vi "Checksum_example.vi"() -> ()   [LabVIEW 2014]
panel:
  in  "String in 2":string
  in  "String in":string
  out "Match?":bool
  out "Checksum":string
  out "Message":string
  out "Example message":string
  out "Calculated checksum":string
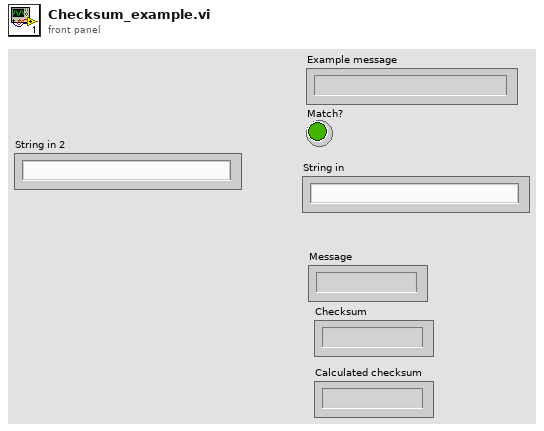
[diagram p1: front panel]
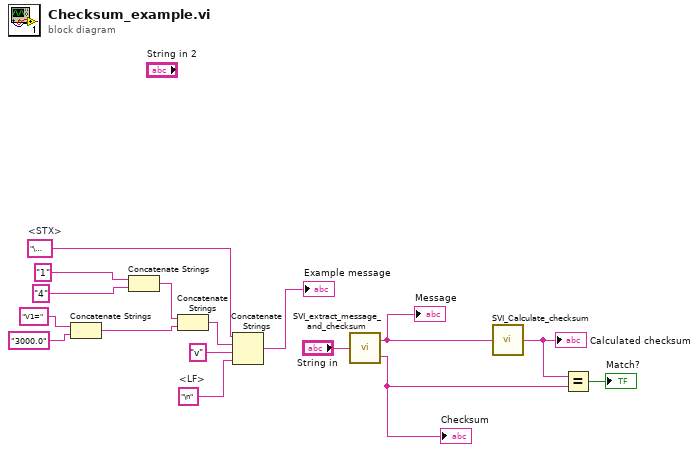
[diagram p0: block diagram]
diagram:
  w8 = "\n"  # <LF>
  w7 = "\u0002"  # <STX>
  n1 = Concatenate Strings("V1=" ("string"), "3000.0" ("string")) -> (w11:string)
  n2 = Concatenate Strings("1" ("string"), "4" ("string")) -> (w12:string)
  n3 = Concatenate Strings(w12, w11) -> (w10:string)
  n4 = Concatenate Strings(w7, w10, "v" ("string"), w8) -> (→"Example message":string)
  n5 = call "SVI_extract_message_and_checksum.vi"("String in"="String in") -> ("Message"=w5:string, "Checksum"=w3:string)
  "Message" <- w5
  "Checksum" <- w3
  n6 = call "SVI_Calculate_checksum.vi"("Message"=w5) -> ("Calculated checksum"=w4:string)
  "Calculated checksum" <- w4
  n7 = Equal?(x=w4, y=w3) -> (x = y?=→"Match?":bool)
